vi "Read Actor Name.vi"(11 "Actor in":refnum<class "Actor.lvclass">) -> (2 "Name":string)   [LabVIEW 2017, in "SequencingModel.lvlib" / "SequencingModel.lvclass"]
uses:
  SequencingModel.lvclass
  <vilib>/ActorFramework/Actor/Actor.lvclass
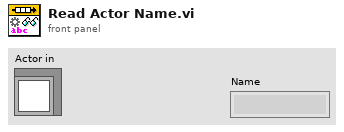
[diagram p1: front panel]
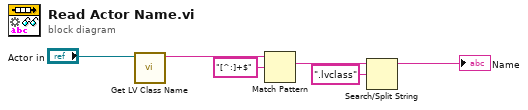
[diagram p0: block diagram]
diagram:
  n1 = call <vilib>:"Get LV Class Name.vi"("object"="Actor in") -> ("class name"=w5:string)  [unwired: 9 in, 1 out]
  n2 = Match Pattern(string=w5, regular expression="[^:]+$") -> (match substring=w3:string)  [unwired: 1 in, 3 out]
  n3 = Search/Split String(string=w3, search string/char (-)=".lvclass") -> (substring before match=→"Name":string)  [unwired: 1 in, 2 out]
